vi "Pololu.Mgr - Move All to Saved Positions.vi"(6 "Ignore Stops":bool, 8 "error in (no error)":errorcluster, 9 "Position Index":i32, 11 "PololuCtrl in":refnum<class "PololuCtrl.lvclass">) -> (0 "error out":errorcluster, 2 "Positions":dbl[](array[numeric]), 3 "PololuCtrl out":refnum<class "PololuCtrl.lvclass">)   [LabVIEW 2018, in "PololuCtrl.lvclass"]
uses:
  PololuCtrl.lvclass
  PololuCtrl.lvclass/PololuCtrl.ctl
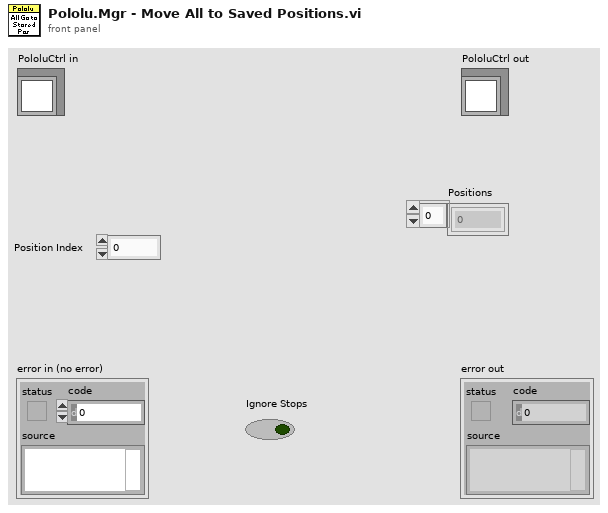
[diagram p1: front panel]
types:
  T1 = typedef "Pololu.Device Config.ctl" = cluster{"Chan":u8, "Accel":u16, "Speed":u16, "Positions":dbl[], "Range Info":T2}
  T2 = typedef "Pololu.Device Range Config.ctl" = cluster{"Min us":dbl, "Max us":dbl, "Min deg":dbl, "Max deg":dbl, "LStopDeg":dbl, "UStopDeg":dbl}
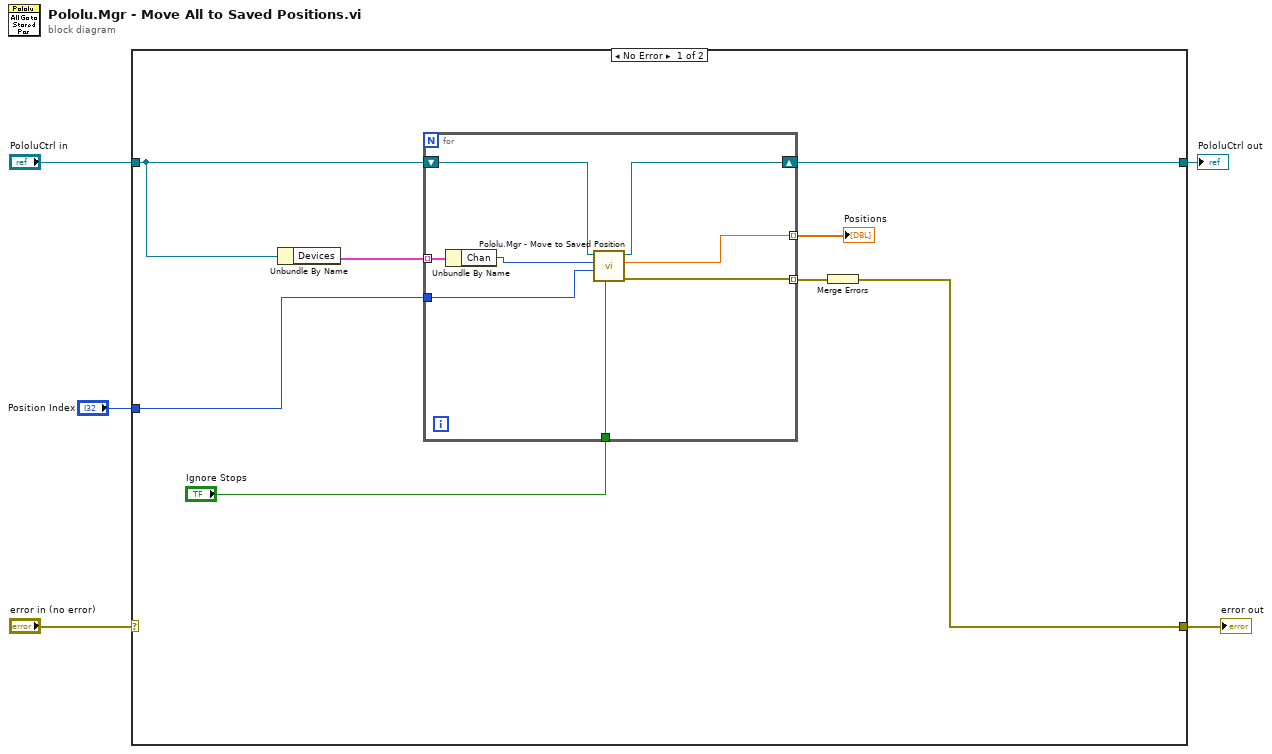
[diagram p0: block diagram]
diagram:
  n1 = case shown="No Error" "error in (no error)" {
    selector: "error in (no error)" -> [_ w23]
    tunnel: [w8 w23] -> w4
    tunnel: [w10 w22] -> w2
    tunnel: "PololuCtrl in" -> [w13 w22]
    tunnel: "Position Index" -> [w11 _]
    frame No Error {
      n2 = Unbundle By Name(w13) -> ("Devices"=w12:T1[])
      n3 = for {
        tunnel: w12 -> [w19] mode=indexing
        tunnel: w11 -> [w20]
        tunnel: [w17] -> w9 mode=indexing
        shift-right: [w16] -> w10
        shift-left: w13 -> [w21]
        tunnel: [w15] -> w7 mode=indexing
        tunnel: "Ignore Stops" -> [w14]
        n4 = Unbundle By Name(w19) -> ("Chan"=w18:u8)
        n5 = call "Pololu.Mgr - Move to Saved Position.vi"("Ignore Stops"=w14, "Position Index"=w20, "Channel"=w18, "PololuCtrl in"=w21) -> ("error out"=w17:errorcluster, "Position(Deg)"=w15:dbl, "PololuCtrl out"=w16:refnum<class "PololuCtrl.lvclass">)  [unwired: 3 in, 2 out]
      }
      "Positions" <- w7
      n6 = Merge Errors(w9) -> (w8:errorcluster)
    }
    frame Error {
    }
  }
  "error out" <- w4
  "PololuCtrl out" <- w2
